vi "Stream Control.vi"(0 "burst size":u32, 1 "reset":bool, 2 "abort":bool, 3 "end continuous mode":bool, 5 "samples per cycle (1)":u32=1, 7 "future trigger":bool, 9 "input valid":bool, 11 "current time":u64, 12 "fifo status":bool, 13 "start trigger":bool) -> (4 "state":T1, 6 "samples processed":u32, 8 "number of malflows":u32, 10 "stream":bool, 14 "fifo ready":bool, 15 "stream start time":u64)   [LabVIEW 2025]
doc: "Controls whether or not data is written to the DMA FIFO for the acquisition stream. If burst size is 0, this will be a continuous stream, started when the start trigger is asserted. If burst size is greater than zero, acquisition will be in bursts of the designated size, initiated each time the internal state machine is idle and a start trigger is received.\n\nThis VI also keeps track of whether or not an overflow occurred in the acquisition stream and counts the number of overflows that have occurred for debugging information.\n\nThe internal state machine returns the number of samples processed since the most recent acquisition began and the current state machine state."
uses:
  Stream Control State.ctl
  <instrlib>/_niInstr/Basic Elements/v1/FPGA/Private/Count Up U32.vi
  <instrlib>/_niInstr/Basic Elements/v1/FPGA/niInstr Basic Elements v1 FPGA.lvlib
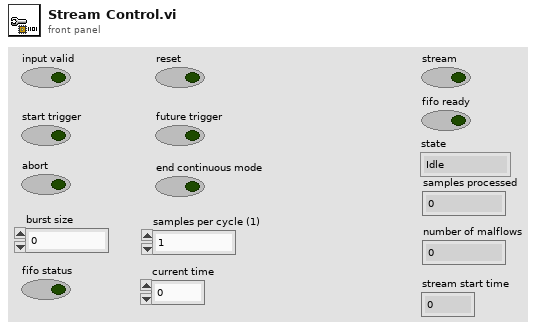
[diagram p1: front panel]
types:
  T1 = typedef "Stream Control State.ctl" = enum16{"Idle", "Active", "WaitForTrigger"}
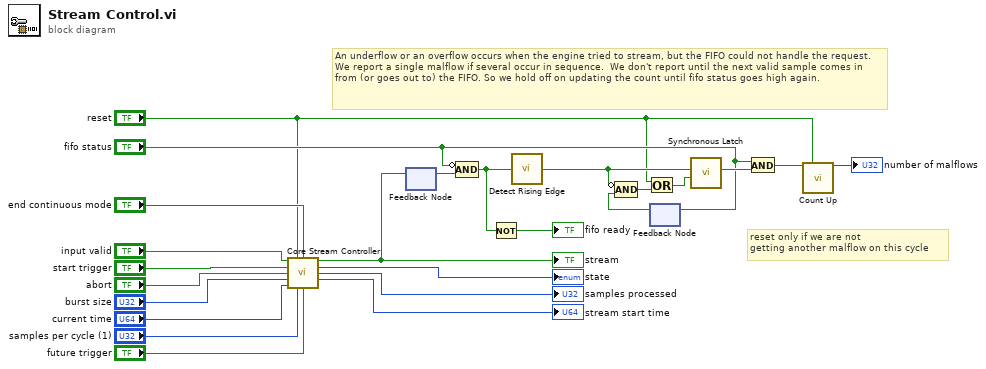
[diagram p0: block diagram]
diagram:
  # "reset only if we are not\ngetting another malflow on this cycle"
  # "An underflow or an overflow occurs when the engine tried to stream, but the FIFO could not handle the request. We report a single malflow if several occur in sequence.  We don't report until the next valid sample comes in from (or goes out to) the FIFO. So we hold off on updating the count until fifo status goes high again."
  n1 = call "Core Stream Controller.vi"("input valid"="input valid", "reset"="reset", "end continuous mode"="end continuous mode", "start trigger"="start trigger", "abort"="abort", "burst size"="burst size", "current time"="current time", "samples per cycle"="samples per cycle (1)", "future trigger"="future trigger") -> ("stream"=w22:bool, "state"=→"state":T1, "samples processed"=→"samples processed":u32, "stream start time"=→"stream start time":u64)  [unwired: 3 in]
  "stream" <- w22
  n2 = feedback #1() -> (w24:bool)  [unwired: 1 in]
  n3 = feedback-in #1(w22) -> ()
  n4 = Compound Arithmetic op=AND(invert "fifo status", w24) -> (w12:bool)
  n5 = Not(x=w12) -> (.not. x?=→"fifo ready":bool)
  n6 = call <instrlib>:"Detect Rising Edge.vi"("signal"=w12) -> ("edge detected"=w8:bool)  [unwired: 14 in]
  n7 = feedback-in #2("fifo status") -> ()
  n8 = feedback #2() -> (w9:bool)  [unwired: 1 in]
  n9 = Compound Arithmetic op=AND(invert w8, w9) -> (w7:bool)
  n10 = Or(x="reset", y=w7) -> (x .or. y?=w6:bool)
  n11 = call <instrlib>:"Synchronous Latch.vi"("clear"=w6, "set"=w8) -> ("out"=w11:bool)  [unwired: 9 in]
  n12 = And(x="fifo status", y=w11) -> (x .and. y?=w4:bool)
  n13 = call-poly <instrlib>:"Count Up.vi"("increment"=w4, "reset"="reset") -> ("count out"=→"number of malflows":u32)  [unwired: 13 in]
